vi "StateSpace_poleplacement.vi"() -> ()   [LabVIEW 2021]
uses:
  <vilib>/addons/Control Design/_Model Construction/Model Typedefs.llb/CD State Space Model (MIMO).ctl
  <vilib>/addons/Control Design/_Model Construction/Model Typedefs.llb/CD General Elements.ctl
  <vilib>/Analysis/Matrix/Datatypes/RealMatrix.ctl
  <vilib>/Analysis/baseanly.llb/Real A x B.vi
  <vilib>/addons/Control Design/_Model Construction/Model Creation.llb/Model Creation SubVI/cd_Create State Space Model.vi
  <vilib>/addons/Control Design/_Time Response Analysis/Time Response.llb/Time Response subVI/cd_Step Response (State-Space).vi
  <vilib>/addons/Control Design/_Dynamic Analysis/Dynamic Analysis.llb/Dynamic Analysis subVI/cd_Poles (State-Space).vi
  <vilib>/addons/Control Design/_Dynamic Analysis/Dynamic Analysis.llb/Dynamic Analysis subVI/cd_Pole-Zero Map (State-Space).vi
  <vilib>/addons/Control Design/_Utility/Model Viewer.llb/Model Viewer SubVI/cd_Draw State-Space Equation (SS).vi
  <vilib>/Analysis/baseanly.llb/Real Inverse Matrix.vi
  <vilib>/Analysis/Matrix/Numeric/Subtract/Subtract - RM,RM.vi
  <vilib>/addons/Control Design/_Time Response Analysis/Time Response.llb/Time Response subVI/cd_Initial Response (State-Space).vi
  <vilib>/addons/Control Design/_Model Construction/NI_LinSys_Model Creation.lvlib
  <vilib>/addons/Control Design/_State-Space Analysis/NI_CD_State-Space Analysis.lvlib
  <vilib>/addons/Control Design/_Utility/NI_CD_Model Viewer.lvlib
  <vilib>/Analysis/NI_AALBase.lvlib
  <vilib>/addons/Control Design/_State Feedback Control/NI_CD_State Feedback Control.lvlib
  <vilib>/addons/Control Design/_Dynamic Analysis/NI_CD_Dynamic Analysis.lvlib
  <vilib>/Analysis/Matrix/NI_Matrix.lvlib
  <vilib>/addons/Control Design/_Time Response Analysis/NI_CD_Time Response.lvlib
  <vilib>/addons/Control Design/_Model Construction/NI_LinSys_Model Typedefs.lvlib
panel:
  out "Step Response uncompansated":cluster{"time":dbl[], dbl[]}[](graph)
  out "Step Response compansated system":cluster{"time":dbl[], dbl[]}[](graph)
  out "Controllable poles":cdb[](array[numeric])=[-3.0000000000000018+0.0i, -4.999999999999998+0.0i] format="%.3f"
  out "Uncompasated system Graph":cluster{"time":dbl[], dbl[]}[](graph)=[{"time"=[0.0, 0.1, 0.2, 0.30000000000000004, 0.4, 0.5, 0.6000000000000001, 0.7000000000000001, 0.8, 0.9, 1.0, 1.1, 1.2000000000000002, 1.3, 1.4000000000000001, 1.5, 1.6, 1.7000000000000002, 1.8, 1.9000000000000001, 2.0, 2.1, 2.2, 2.3000000000000003, 2.4000000000000004, 2.5, 2.6, 2.7, 2.8000000000000003, 2.9000000000000004, 3.0, 3.1, 3.2, 3.3000000000000003, 3.4000000000000004, 3.5, 3.6, 3.7, 3.8000000000000003, 3.9000000000000004, 4.0, 4.1000000000000005, 4.2, 4.3, 4.4, 4.5, 4.6000000000000005, 4.7, 4.800000000000001, 4.9, 5.0, 5.1000000000000005, 5.2, 5.300000000000001, 5.4, 5.5, 5.6000000000000005, 5.7, 5.800000000000001, 5.9, 6.0, 6.1000000000000005, 6.2, 6.300000000000001, 6.4, 6.5, 6.6000000000000005, 6.7, 6.800000000000001, 6.9, 7.0, 7.1000000000000005, 7.2, 7.300000000000001, 7.4, 7.5, 7.6000000000000005, 7.7, 7.800000000000001, 7.9, 8.0], [10.0, 11.631574129098434, 12.639628742049286, 13.168379744446929, 13.332932917907842, 13.224843153360961, 12.916639086393909, 12.46550323340715, 11.916263024848233, 11.303819742975477, 10.655119149758503, 9.99074859705244, 9.326229877805062, 8.673064374929915, 8.039576678907217, 7.4315943549008345, 6.8529946004348465, 6.306142863299272, 5.792243855444399, 5.311621613220188, 4.863942162802272, 4.448389825504766, 4.063806137401149, 3.708798676573012, 3.3818257201057897, 3.0812615349832955, 2.8054461959504544, 2.5527230813115454, 2.3214665935141765, 2.1101021598949696, 1.9171201694145295, 1.7410851766534094, 1.5806414409394054, 1.4345156549231428, 1.3015175439776825, 1.1805388779260912, 1.0705513236403914, 0.9706034759796801, 0.8798173312433991, 0.7973844084627771, 0.7225616767122883, 0.6546674089712832, 0.5930770530937413, 0.537219186678009, 0.4865716038698731, 0.44065756740709205, 0.399042247730231, 0.36132936210113453, 0.32715801986607657, 0.2961997748540095, 0.2681558820705454, 0.242754753060103, 0.21974960234018018, 0.19891627598446493, 0.18005125260217292, 0.16296980651485665, 0.1475043227773481, 0.13350275375357443, 0.12082720718294636, 0.1093526560132836, 0.09896576069605557, 0.08956379511121978, 0.08105366779060427, 0.073351030624133, 0.06637946774979712, 0.06006975783689428, 0.05435920346598904, 0.049191021783575664, 0.04451379106139409, 0.040280948217810975, 0.03645033276060811, 0.03298377298660477, 0.029846710623989584, 0.027007860428650516, 0.024438901547043673, 0.022114197736298684, 0.02001054378850781, 0.01810693574174538, 0.01638436267660179, 0.014825618095180057, 0.01341512906085916]}, {"time"=[0.0, 0.1, 0.2, 0.30000000000000004, 0.4, 0.5, 0.6000000000000001, 0.7000000000000001, 0.8, 0.9, 1.0, 1.1, 1.2000000000000002, 1.3, 1.4000000000000001, 1.5, 1.6, 1.7000000000000002, 1.8, 1.9000000000000001, 2.0, 2.1, 2.2, 2.3000000000000003, 2.4000000000000004, 2.5, 2.6, 2.7, 2.8000000000000003, 2.9000000000000004, 3.0, 3.1, 3.2, 3.3000000000000003, 3.4000000000000004, 3.5, 3.6, 3.7, 3.8000000000000003, 3.9000000000000004, 4.0, 4.1000000000000005, 4.2, 4.3, 4.4, 4.5, 4.6000000000000005, 4.7, 4.800000000000001, 4.9, 5.0, 5.1000000000000005, 5.2, 5.300000000000001, 5.4, 5.5, 5.6000000000000005, 5.7, 5.800000000000001, 5.9, 6.0, 6.1000000000000005, 6.2, 6.300000000000001, 6.4, 6.5, 6.6000000000000005, 6.7, 6.800000000000001, 6.9, 7.0, 7.1000000000000005, 7.2, 7.300000000000001, 7.4, 7.5, 7.6000000000000005, 7.7, 7.800000000000001, 7.9, 8.0], [20.0, 12.930348463241515, 7.469972639020698, 3.2959693383748556, 0.14693600560989006, -2.1884599182165796, -3.880812729026752, -5.06759431515791, -5.859367485007591, -6.344853096326978, -6.595060652659299, -6.6666538461816796, -6.604691279122022, -6.4448570284993085, -6.215274800150157, -5.937982303864459, -5.63012848108346, -5.304944764489141, -4.9725321820253185, -4.6404984575349575, -4.314472996140019, -3.998522520890238, -3.6954859403089273, -3.4072436042338596, -3.1349333086350644, -2.879123125010625, -2.63994926332754, -2.4172256530330873, -2.210530682019622, -2.0192755175336385, -1.8427576041144909, -1.6802022575644966, -1.5307947227441527, -1.3937046137966767, -1.2681042895423134, -1.1531824189594344, -1.048153749389073, -0.9522658931457775, -0.8648037882401676, -0.7850923590933723, -0.7124977978752034, -0.6464278018721108, -0.5863310333683689, -0.5316960128679757, -0.48204961161700366, -0.43695527328448724, -0.39601106567511446, -0.3588476401344323, -0.3251261577713481, -0.29453622687104175, -0.2667938841776688, -0.2416396434995774, -0.21883662784992652, -0.19816879569251855, -0.17943926749983669, -0.16246875549114836, -0.1470940968953769, -0.13316688920829603, -0.12055222455085834, -0.1091275192758308, -0.09878143432545529, -0.08941288144300605, -0.08093011012937786, -0.07324987016710853, -0.06629664457263573, -0.060001947954684595, -0.054303685430061366, -0.049145567460211176, -0.04447657620899522, -0.04025047927368076, -0.036425386899034885, -0.03296334904257273, -0.0298299889129114, -0.026994169849546713, -0.024427692648903935, -0.02210502066668356, -0.020003030239390766, -0.018100784168018493, -0.016379326194011758, -0.014821494571996252, -0.013411753005617545]}]
  out "Companstaed system Graph":cluster{"time":dbl[], dbl[]}[](graph)=[{"time"=[0.0, 0.040000000000000015, 0.08000000000000003, 0.12000000000000005, 0.16000000000000006, 0.20000000000000007, 0.2400000000000001, 0.2800000000000001, 0.3200000000000001, 0.36000000000000015, 0.40000000000000013, 0.44000000000000017, 0.4800000000000002, 0.5200000000000002, 0.5600000000000002, 0.6000000000000002, 0.6400000000000002, 0.6800000000000003, 0.7200000000000003, 0.7600000000000002, 0.8000000000000003, 0.8400000000000003, 0.8800000000000003, 0.9200000000000004, 0.9600000000000004, 1.0000000000000004, 1.0400000000000005, 1.0800000000000003, 1.1200000000000003, 1.1600000000000004, 1.2000000000000004, 1.2400000000000004, 1.2800000000000005, 1.3200000000000005, 1.3600000000000005, 1.4000000000000006, 1.4400000000000006, 1.4800000000000006, 1.5200000000000005, 1.5600000000000005, 1.6000000000000005, 1.6400000000000006, 1.6800000000000006, 1.7200000000000006, 1.7600000000000007, 1.8000000000000007, 1.8400000000000007, 1.8800000000000008, 1.9200000000000008, 1.9600000000000006, 2.000000000000001, 2.040000000000001, 2.080000000000001, 2.120000000000001, 2.1600000000000006, 2.2000000000000006, 2.2400000000000007, 2.2800000000000007, 2.3200000000000007, 2.3600000000000008, 2.400000000000001, 2.440000000000001, 2.480000000000001, 2.520000000000001, 2.560000000000001, 2.600000000000001, 2.640000000000001, 2.680000000000001], [10.0, 10.573946458150962, 10.773973986438378, 10.698380510135413, 10.424194610284374, 10.01142123400485, 9.506473660793937, 8.944944221477607, 8.353838059262515, 7.753371192033185, 7.158415336011735, 6.579656609746395, 6.024522721638928, 5.497923036668398, 5.00283759574888, 4.540784378558912, 4.112188575103081, 3.716673131736738, 3.3532861751498584, 3.0206779386396567, 2.71723739291107, 2.44119681572168, 2.1907109368967896, 1.9639159989715755, 1.7589730229691702, 1.5740987178980927, 1.4075867841702232, 1.2578218048992238, 1.1232874701537698, 1.0025705175118864, 0.8943614812385753, 0.7974531086917909, 0.7107371152487945, 0.633199799267706, 0.5639169191485611, 0.5020481395778535, 0.44683127877611206, 0.3975765291630628, 0.35366077718392025, 0.314522111572769, 0.27965458101813623, 0.24860324038829504, 0.2209595080356564, 0.19635684415620624, 0.17446675086708358, 0.1549950878892753, 0.13767869292723633, 0.12228229257883094, 0.1085956875332833, 0.09643119464048441, 0.08562132793925982, 0.0760167007393849, 0.06748413122436867, 0.05990493467171246, 0.05317338619107655, 0.04719533879441979, 0.04188698258688908, 0.03717373186632111, 0.03298922791552412, 0.029274446245372086, 0.025976897984350388, 0.023049916002251727, 0.020452017196421146, 0.018146333155121826, 0.016100102143056745, 0.014284216029117905, 0.012672816397387033, 0.011242934651361997]}, {"time"=[0.0, 0.040000000000000015, 0.08000000000000003, 0.12000000000000005, 0.16000000000000006, 0.20000000000000007, 0.2400000000000001, 0.2800000000000001, 0.3200000000000001, 0.36000000000000015, 0.40000000000000013, 0.44000000000000017, 0.4800000000000002, 0.5200000000000002, 0.5600000000000002, 0.6000000000000002, 0.6400000000000002, 0.6800000000000003, 0.7200000000000003, 0.7600000000000002, 0.8000000000000003, 0.8400000000000003, 0.8800000000000003, 0.9200000000000004, 0.9600000000000004, 1.0000000000000004, 1.0400000000000005, 1.0800000000000003, 1.1200000000000003, 1.1600000000000004, 1.2000000000000004, 1.2400000000000004, 1.2800000000000005, 1.3200000000000005, 1.3600000000000005, 1.4000000000000006, 1.4400000000000006, 1.4800000000000006, 1.5200000000000005, 1.5600000000000005, 1.6000000000000005, 1.6400000000000006, 1.6800000000000006, 1.7200000000000006, 1.7600000000000007, 1.8000000000000007, 1.8400000000000007, 1.8800000000000008, 1.9200000000000008, 1.9600000000000006, 2.000000000000001, 2.040000000000001, 2.080000000000001, 2.120000000000001, 2.1600000000000006, 2.2000000000000006, 2.2400000000000007, 2.2800000000000007, 2.3200000000000007, 2.3600000000000008, 2.400000000000001, 2.440000000000001, 2.480000000000001, 2.520000000000001, 2.560000000000001, 2.600000000000001, 2.640000000000001, 2.680000000000001], [20.0, 9.214698279446193, 1.1940803424668092, -4.654559725704944, -8.806135624992068, -11.640291643442454, -13.459710386771722, -14.50498446735251, -14.966688278054786, -14.99516916502024, -14.708481846204577, -14.198811911122496, -13.537670500446163, -12.780090199288503, -11.968009655985743, -11.132999717283537, -10.298455526390933, -9.48135589719391, -8.693672403084946, -7.943495223110688, -7.235930234296497, -6.573811606141151, -5.958265815536942, -5.389156209683041, -4.865431716456503, -4.385398803739999, -3.946932131472626, -3.547636367567033, -3.184969224637159, -2.856333815266865, -2.559146834882405, -2.290887794260583, -2.049133482087684, -1.8315809959257208, -1.636062000053441, -1.460550320455833, -1.3031645459095005, -1.1621669494327083, -1.035959759879729, -0.9230795857693166, -0.822190611659282, -0.732077042666277, -0.6516351578980257, -0.5798652427852388, -0.5158635988464759, -0.45881477346349103, -0.4079841086898536, -0.36271067445866056, -0.3224006257753066, -0.2865210039498438, -0.25459398732965466, -0.22619158628394787, -0.20093076952268538, -0.17846900352856185, -0.15850018340267072, -0.14075093134374678, -0.12497723795738293, -0.11096142135683354, -0.09850937935975977, -0.08744811084036223, -0.07762348333538459, -0.06889822522639946, -0.061150122153886516, -0.0542703987036584, -0.04816226780056827, -0.04273963161700457, -0.037925919132281924, -0.03365304674847876]}]
  in  "Initial Conditions":dbl[](array[numeric])=[10.0, 20.0] format="%.3f"
  out "Open Loop Poles":cdb[](array[numeric])=[-1.0+0.0i, -2.0+0.0i] format="%.3f"
  out "Pole-Zero Map":cluster{dbl[], dbl[]}[](graph)=[{[-1.0, -2.0], [0.0, 0.0]}, {[], []}]
  out "K (Gain)":dbl[][](array[numeric])=[[6.500000000000002, 2.5000000000000004]] format="%.2f"
  in  "Gain Type":u16(ring) items=["Controller Gain", "Observer Gain (Predictive)", "Observer Gain (Current)"]
  in  "Desired Poles":cdb[](array[numeric])=[-3.0+0.0i, -5.0+0.0i] format="%.2f"
  out "Transformation Matrix(T)":T1=[[2.0, 0.0], [0.0, 2.0]]
  out "Equation":picture
  in  "Form Type":u16(ring)=1 items=["Modal"=0, "Companion"=5, "Controllability"=1, "Controller Companion"=2, "Observability"=3, "Observer Companion"=4]
  out "Transformation Matrix inverse (T')":dbl[][](array[numeric])=[[0.5, 0.0], [-0.0, 0.5]] format="%.2f"
  out "new Transformed Model":T2={"properties"={"Model name"="System Model", "Input names"=["u0"], "Output names"=["y0"], "Input Delays"=[0.0], "Output Delays"=[0.0], "Sampling Time"=0.0, "Notes"=""}, "A"=[[0.0, 1.0], [-2.0, -3.0]], "B"=[[0.0], [1.0]], "C"=[[2.0, 0.0]], "D"=[[0.0]], "StateNames"=["x0", "x1"], "Transport Delay"=[[0.0]]} {"Transport Delay" format="%.2f"; "D" format="%#.2g"; "C" format="%#.2g"; "B" format="%#.2g"; "A" format="%#.2g"; "properties"."Sampling Time" format="%#.6p"; "properties"."Output Delays" format="%.4f"; "properties"."Input Delays" format="%.4f"}
  out "Is Controllable?":bool=TRUE
  out "Controllability Matrix (M)":dbl[][](array[numeric])=[[0.0, 2.0], [2.0, -6.0]] format="%.2f"
  in  "D":dbl[][](array[numeric])=[[0.0]] format="%#.5g"
  in  "C":dbl[][](array[numeric])=[[1.0, 0.0]] format="%#.5g"
  in  "B":dbl[][](array[numeric])=[[0.0], [2.0]] format="%#.5g"
  in  "A":dbl[][](array[numeric])=[[0.0, 1.0], [-2.0, -3.0]] format="%#.5g"
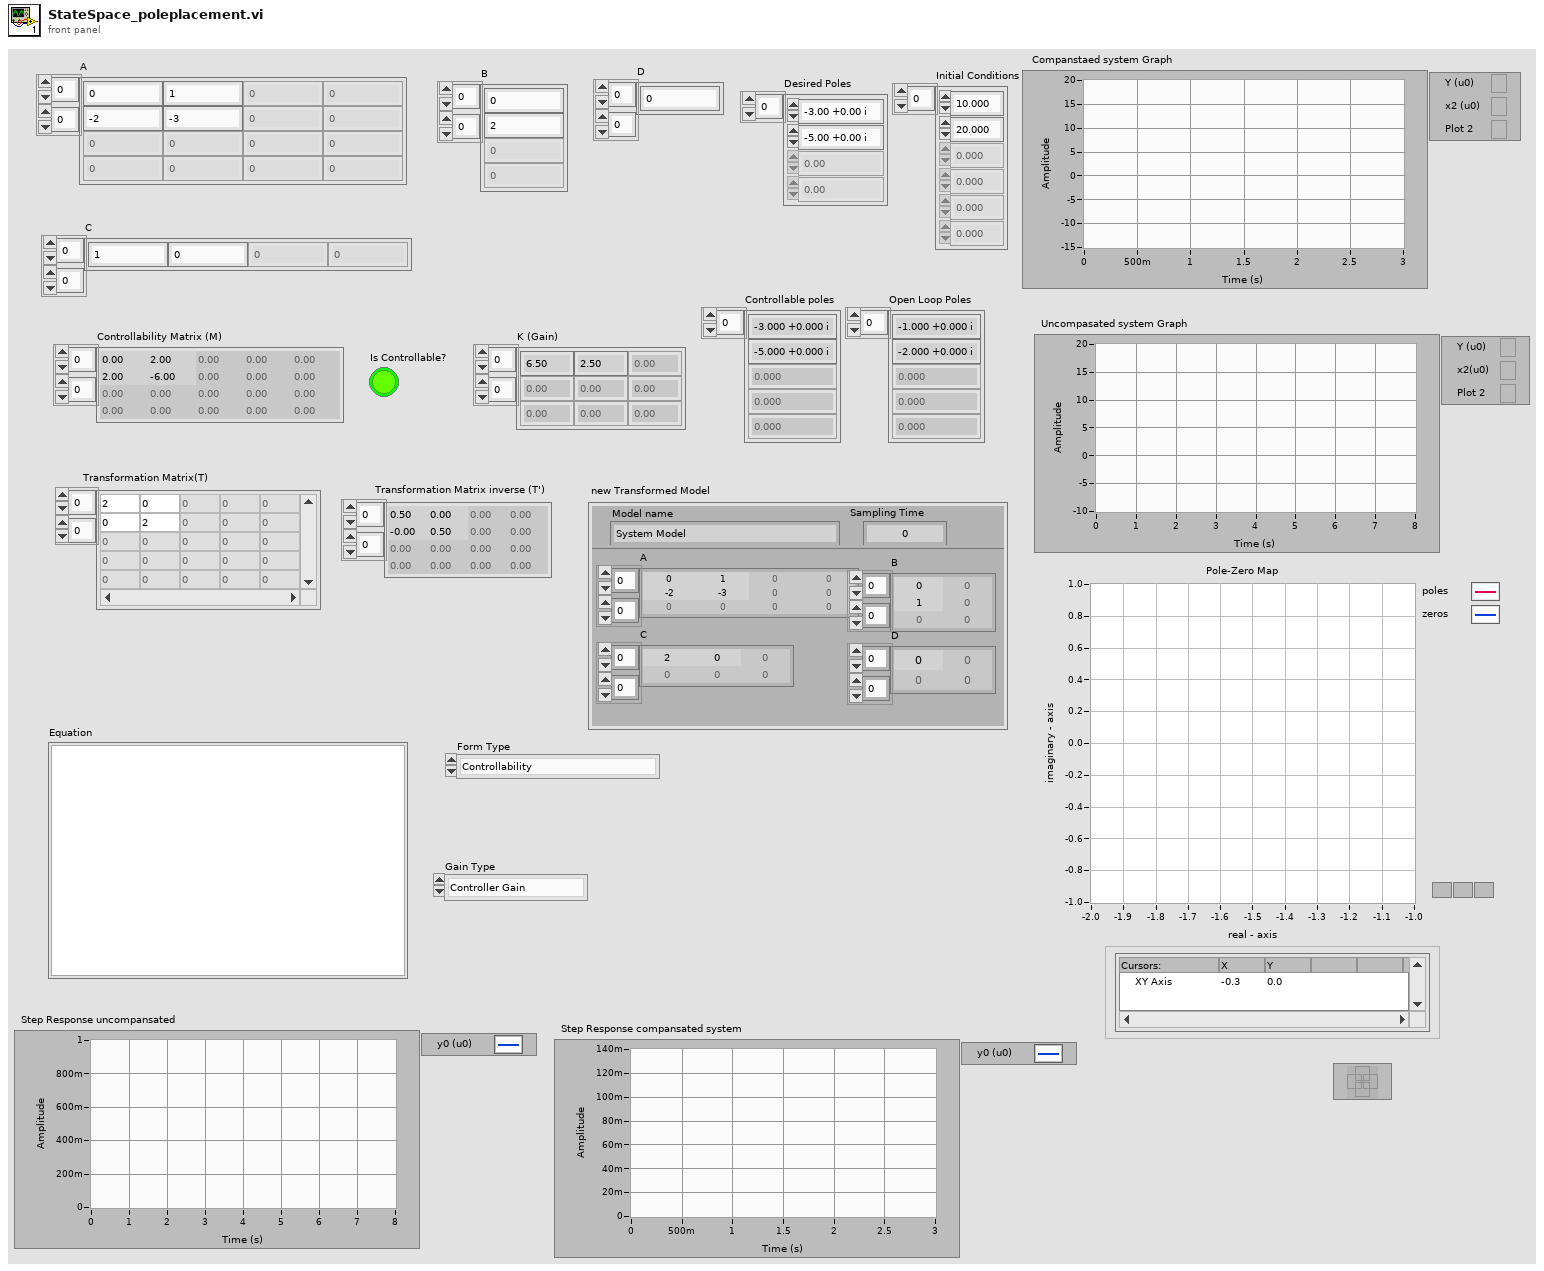
[diagram p1: front panel]
types:
  T1 = typedef "NI_Matrix.lvlib/RealMatrix.ctl" = dbl[][]
  T2 = typedef "NI_LinSys_Model Typedefs.lvlib/CD State Space Model (MIMO).ctl" = cluster{"properties":T3, "A":dbl[][], "B":dbl[][], "C":dbl[][], "D":dbl[][], "StateNames":string[], "Transport Delay":dbl[][]}
  T3 = typedef "NI_LinSys_Model Typedefs.lvlib/CD General Elements.ctl" = cluster{"Model name":string, "Input names":string[], "Output names":string[], "Input Delays":dbl[], "Output Delays":dbl[], "Sampling Time":dbl, "Notes":string}
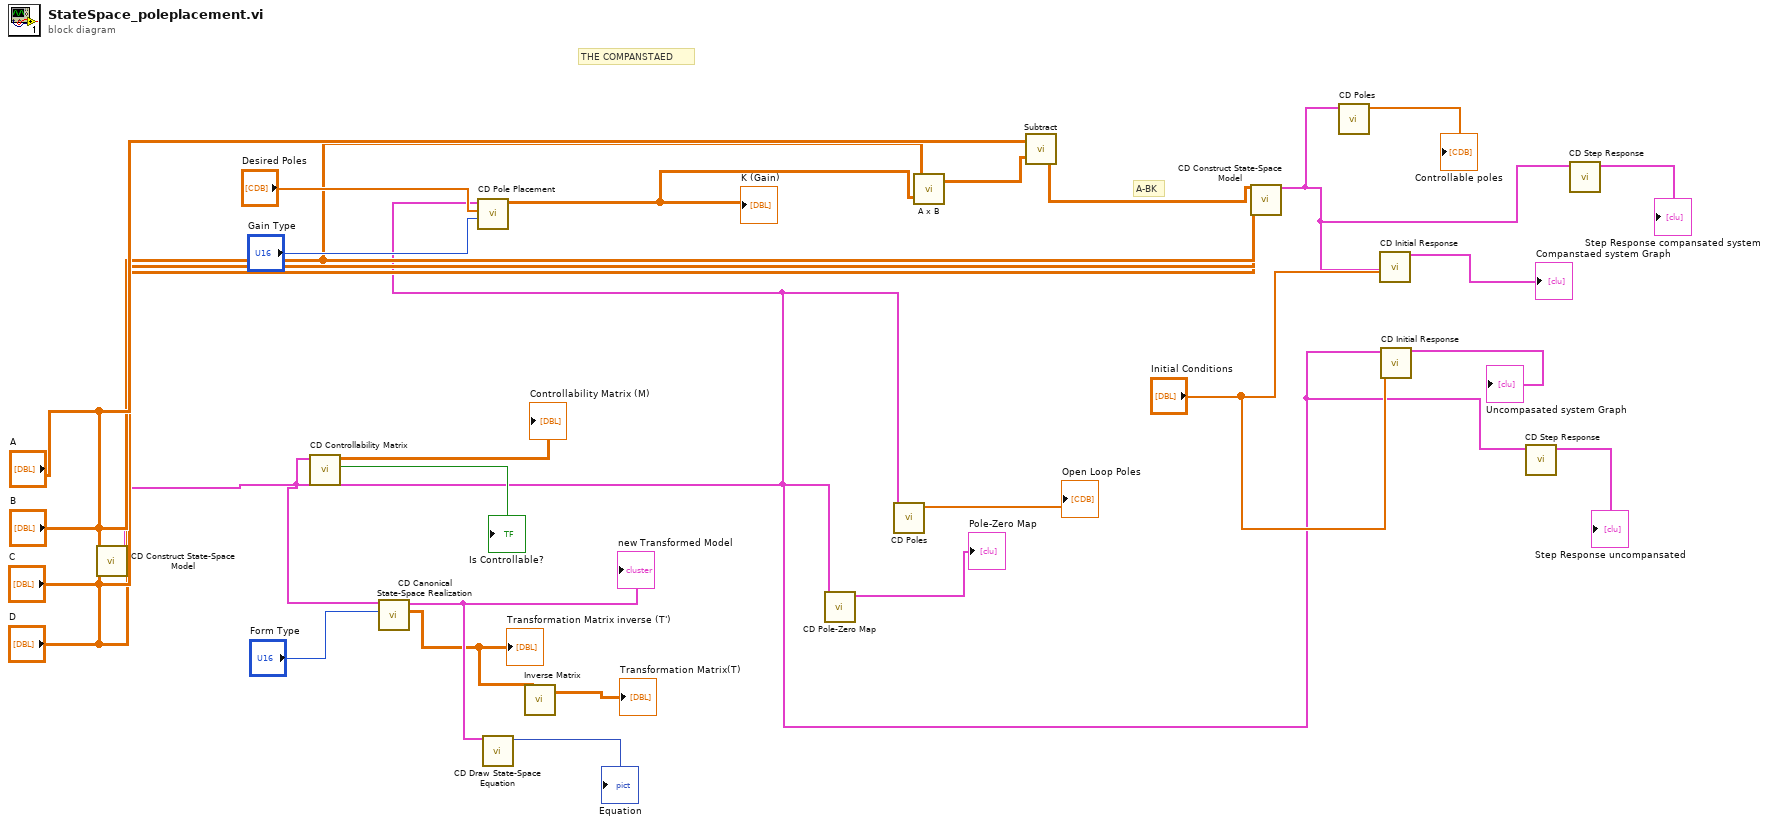
[diagram p0: block diagram]
diagram:
  # "THE COMPANSTAED"
  # "A-BK"
  n1 = call-poly <vilib>:"CD Construct State-Space Model.vi"("A"="A", "B"="B", "C"="C", "D"="D") -> ("State-Space Model"=w2:T2)  [unwired: 10 in, 1 out]
  n2 = call <vilib>:"CD Controllability Matrix.vi"("State-Space Model"=w2) -> ("Is Controllable?"=→"Is Controllable?":bool, "Controllability Matrix"=→"Controllability Matrix (M)":dbl[][])  [unwired: 7 in, 2 out]
  n3 = call <vilib>:"CD Canonical State-Space Realization.vi"("Form Type"="Form Type", "State-Space Model"=w2) -> ("Transformation Matrix (T)"=w21:dbl[][], "Transformed Model"=w23:T2)  [unwired: 7 in, 1 out]
  "new Transformed Model" <- w23
  "Transformation Matrix inverse (T')" <- w21
  n4 = call <vilib>:"CD Pole Placement.vi"("Gain Type"="Gain Type", "Poles"="Desired Poles", "State-Space Model"=w2) -> ("Gain"=w15:dbl[][])  [unwired: 6 in, 2 out]
  "K (Gain)" <- w15
  n5 = call-poly <vilib>:"CD Draw State-Space Equation.vi"("State-Space Model"=w23) -> ("Equation"=→"Equation":picture)  [unwired: 8 in, 2 out]
  n6 = call-poly <vilib>:"Inverse Matrix.vi"("Input Matrix"=w21) -> ("Inverse Matrix"=→"Transformation Matrix(T)":T1)  [unwired: 1 in, 1 out]
  n7 = call-poly <vilib>:"CD Pole-Zero Map.vi"("State-Space Model"=w2) -> ("Pole-Zero Map"=→"Pole-Zero Map":cluster{dbl[], dbl[]}[])  [unwired: 7 in, 3 out]
  n8 = call-poly <vilib>:"CD Poles.vi"("State-Space Model"=w2) -> ("Poles"=→"Open Loop Poles":cdb[])  [unwired: 9 in, 1 out]
  n9 = call-poly <vilib>:"A x B.vi"("B"=w15, "A"="B") -> ("A x B"=w14:T1)  [unwired: 1 out]
  n10 = call-poly <vilib>:"Subtract.vi"("Real Matrix B"=w14, "Real Matrix A"="A") -> ("A - B"=w12:T1)
  n11 = call-poly <vilib>:"CD Construct State-Space Model.vi"("A"=w12, "B"="B", "C"="C", "D"="D") -> ("State-Space Model"=w4:T2)  [unwired: 10 in, 1 out]
  n12 = call-poly <vilib>:"CD Poles.vi"("State-Space Model"=w4) -> ("Poles"=→"Controllable poles":cdb[])  [unwired: 9 in, 1 out]
  n13 = call-poly <vilib>:"CD Initial Response.vi"("Initial Conditions"="Initial Conditions", "State-Space Model"=w4) -> ("State Trajectory Graph"=→"Companstaed system Graph":cluster{"time":dbl[], dbl[]}[])  [unwired: 6 in, 3 out]
  n14 = call-poly <vilib>:"CD Initial Response.vi"("Initial Conditions"="Initial Conditions", "State-Space Model"=w2) -> ("State Trajectory Graph"=→"Uncompasated system Graph":cluster{"time":dbl[], dbl[]}[])  [unwired: 6 in, 3 out]
  n15 = call-poly <vilib>:"CD Step Response.vi"("State-Space Model"=w2) -> ("Step Response Graph"=→"Step Response uncompansated":cluster{"time":dbl[], dbl[]}[])  [unwired: 7 in, 3 out]
  n16 = call-poly <vilib>:"CD Step Response.vi"("State-Space Model"=w4) -> ("Step Response Graph"=→"Step Response compansated system":cluster{"time":dbl[], dbl[]}[])  [unwired: 7 in, 3 out]
